vi "WakeUp.vi"(8 "error in (no error)":errorcluster, 11 "PCA in":refnum<class "PCA.lvclass">) -> (0 "error out":errorcluster, 3 "PCA out":refnum<class "PCA.lvclass">)   [LabVIEW 2022 SP3, in "PCA9685.lvlib" / "PCA.lvclass"]
uses:
  PCA.lvclass
  PCA.lvclass/PCA.ctl
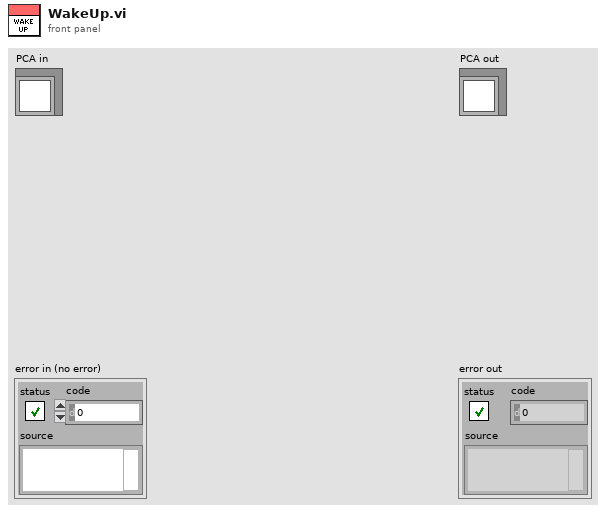
[diagram p1: front panel]
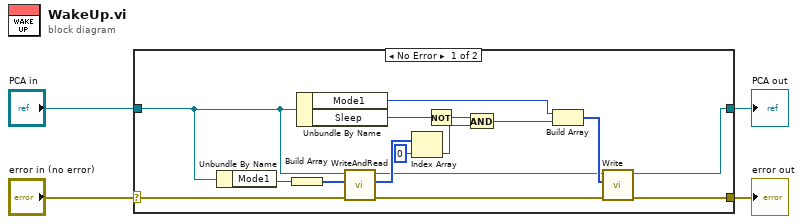
[diagram p0: block diagram]
diagram:
  n1 = case shown="No Error" "error in (no error)" {
    selector: "error in (no error)" -> [w10 w22]
    tunnel: [w9 w22] -> w3
    tunnel: [w5 w21] -> w1
    tunnel: "PCA in" -> [w8 w21]
    frame No Error {
      n2 = Unbundle By Name(w8) -> ("Mode1"=w20:u8)
      n3 = Build Array(w20) -> (w19:u8[])
      n4 = Unbundle By Name(w8) -> ("Mode1"=w13:u8, "Sleep"=w7:u8)
      n5 = call "WriteAndRead.vi"("error in (no error)"=w10, "Data"=w19, "PCA in"=w8) -> ("error out"=w15:errorcluster, "Data 2"=w17:u8[], "PCA out"=w11:refnum<class "PCA.lvclass">)  [unwired: 6 in]
      n6 = Index Array(array=w17, index=0) -> (element=w18:u8)
      n7 = Not(x=w7) -> (.not. x?=w6:u8)
      n8 = And(x=w6, y=w18) -> (x .and. y?=w14:u8)
      n9 = Build Array(w13, w14) -> (w12:u8[])
      n10 = call "Write.vi"("error in (no error)"=w15, "Data"=w12, "PCA in"=w11) -> ("error out"=w9:errorcluster, "PCA out"=w5:refnum<class "PCA.lvclass">)  [unwired: 7 in]
    }
    frame Error {
    }
  }
  "error out" <- w3
  "PCA out" <- w1
